vi "CAPTH-Get Defaults.vi"(7 "User":string) -> (4 "Params":T1={"Stimulus"={"EAR"=enum."RIGHT", "HI FREQ"=18.0, "LO FREQ"=5.0, "FREQ STEP"=8, "Rep Rate (/s)"=20.0, "Alternate Polarity"=TRUE, "# CYCLES"=1, "Duration (ms)"=0.0, "Ramp (ms)"=0.0}, "Response"={"Averages (3dB steps)"=12, "Time Window (ms)"=8.5, "dt (us)"=10.0, "Grass gain"=1000.0, "CRITERION (mV)"=60.0, "CEILING (dB atten)"=6.0, "Use previous"=FALSE, "Save avgs"=FALSE, "Save raw"=FALSE, "Save history"=FALSE, "CEILING (dB SPL)"=6.0}} {"Response"."CRITERION (mV)" format="%.2f"; "Response"."Time Window (ms)" format="%.2f"})   [LabVIEW 2020]
uses:
  Typedefs/CAPTH-Parameters.ctl
  Typedefs/CAPTH-Stimulus.ctl
  Typedefs/CAPTH-Response.ctl
panel:
  in  "Defaults":T1={"Stimulus"={"EAR"=enum."RIGHT", "HI FREQ"=18.0, "LO FREQ"=5.0, "FREQ STEP"=8, "Rep Rate (/s)"=20.0, "Alternate Polarity"=TRUE, "# CYCLES"=1, "Duration (ms)"=0.0, "Ramp (ms)"=0.0}, "Response"={"Averages (3dB steps)"=12, "Time Window (ms)"=8.5, "dt (us)"=10.0, "Grass gain"=1000.0, "CRITERION (mV)"=60.0, "CEILING (dB atten)"=6.0, "Use previous"=FALSE, "Save avgs"=FALSE, "Save raw"=FALSE, "Save history"=FALSE, "CEILING (dB SPL)"=inf}} {"Response"."CRITERION (mV)" format="%.2f"; "Response"."Time Window (ms)" format="%.2f"}
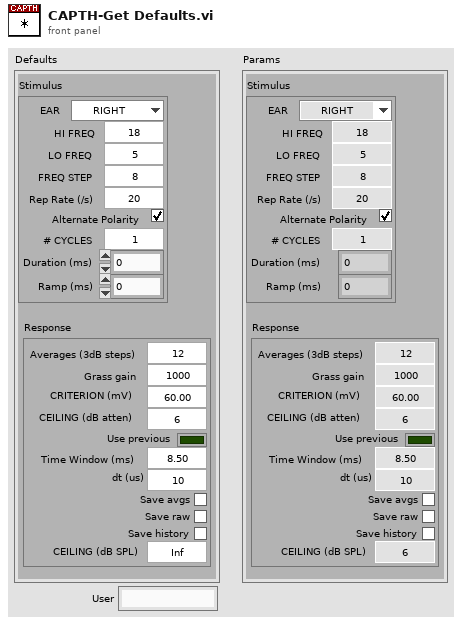
[diagram p1: front panel]
types:
  T1 = typedef "CAPTH-Parameters.ctl" = cluster{"Stimulus":T2, "Response":T3}
  T2 = typedef "CAPTH-Stimulus.ctl" = cluster{"EAR":enum16{"RIGHT", "LEFT\n", "ALTERNATE"}, "HI FREQ":dbl, "LO FREQ":dbl, "FREQ STEP":u8, "Rep Rate (/s)":dbl, "Alternate Polarity":bool, "# CYCLES":u8, "Duration (ms)":dbl, "Ramp (ms)":dbl}
  T3 = typedef "CAPTH-Response.ctl" = cluster{"Averages (3dB steps)":i32, "Time Window (ms)":dbl, "dt (us)":dbl, "Grass gain":dbl, "CRITERION (mV)":dbl, "CEILING (dB atten)":dbl, "Use previous":bool, "Save avgs":bool, "Save raw":bool, "Save history":bool, "CEILING (dB SPL)":dbl}
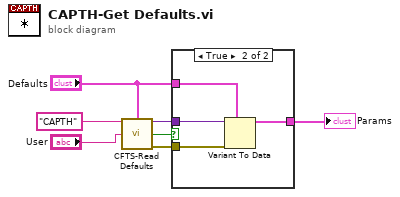
[diagram p0: block diagram]
diagram:
  n1 = call "CFTS-Read Defaults.vi"("AppName"="CAPTH", "Type of anything"="Defaults", "User"="User") -> ("Anything"=w4:variant, "Found?"=w3:bool, "error out"=w5:errorcluster)  [unwired: 10 in]
  n2 = case shown="True" w3 {
    tunnel: w5 -> [_ w12]
    tunnel: w4 -> [_ w11]
    tunnel: "Defaults" -> [w8 w10]
    tunnel: [w8 w9] -> w1
    frame False {
    }
    frame True {
      n3 = Variant To Data(error in=w12, type=w10, Variant=w11) -> (data=w9:T1)  [unwired: 1 out]
    }
  }
  "Params" <- w1
